vi "gyro -- launch async pll.vi"(8 "pll parameters":T1={"PID parameters"={"I (sec)"=0.004634123928756344, "P (sec)"=0.008980860327047186}, "PID mode"=enum."normal", "lorentzian"={"A (VHz)"=0.0007250653088846297, "f (Hz)"=45017.43809779818, "G (Hz)"=34.46000858512321, "phi(rad)"=-1.525051560312372, "Q"=1306.3675821959234, "Norm  Ampl"=nan, "bg (V)"=7.168586400274938e-06+0.00021232547061132137i, "4corners"={"z (-pi/2)"=-1.288800856206544e-05+0.00019034453621736468i, "z(inf)"=7.168586400274938e-06+0.00021232547061132137i, "z (pi/2)"=-1.4812347993681768e-05+0.00023238206557366173i, "z center"=-1.3850178277873603e-05+0.0002113633008955132i, "z(0)"=-3.486894295602214e-05+0.00021040113117970505i, "radius"=2.1040775631078887e-05}}, "plot hist time (sec)"=1.0, "dt (sec)"=0.001, "visc hist time (sec)"=2.0, "time int ave time (sec)"=0.3, "PLL limits (Hz)"=5000.0, "PLL ON"=FALSE} {"PLL limits (Hz)" format="%#.2f"; "time int ave time (sec)" format="%#_10f"; "visc hist time (sec)" format="%#_10f"; "dt (sec)" format="%#_10f"; "plot hist time (sec)" format="%#_10f"; "lorentzian"."bg (V)" format="%#9_9f"; "lorentzian"."Q" format="%#9_9f"; "lorentzian"."phi(rad)" format="%#9_9f"; "lorentzian"."G (Hz)" format="%#9_9f"; "lorentzian"."f (Hz)" format="%#9_9f"; "PID parameters"."P (sec)" scale=0.01..10.0; "PID parameters"."I (sec)" scale=0.01..10.0}, 10 "talkback event":refnum<user-event>) -> (2 "reference out":refnum<vi>)   [LabVIEW 2018]
uses:
  pll talkback message type.ctl
  pll talkto event type.ctl
  pid -- parameters.ctl
  PID - mode.ctl
  circle corners.ctl
  lorentzian.ctl
  pll parameters.ctl
  pll talkback event.ctl
  pll talkto event.ctl
panel:
  in  "pll talkto event":refnum<vi>
  in  "set step !":dbl(slide)=7372.340425531916 min=0.0 max=16000.0 scale=0.0..16500.0 scale format="%^#6_6g"
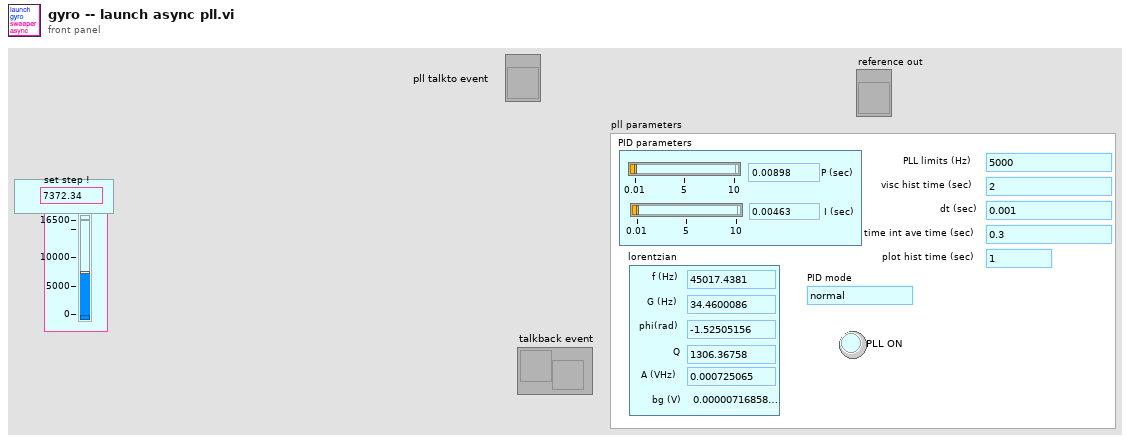
[diagram p1: front panel]
types:
  T1 = typedef "pll parameters.ctl" = cluster{"PID parameters":T2, "PID mode":T3, "lorentzian":T4, "plot hist time (sec)":dbl, "dt (sec)":dbl, "visc hist time (sec)":dbl, "time int ave time (sec)":dbl, "PLL limits (Hz)":dbl, "PLL ON":bool}
  T2 = typedef "pid -- parameters.ctl" = cluster{"I (sec)":dbl, "P (sec)":dbl}
  T3 = typedef "PID - mode.ctl" = enum16{"normal", "heat"}
  T4 = typedef "lorentzian.ctl" = cluster{"A (VHz)":dbl, "f (Hz)":dbl, "G (Hz)":dbl, "phi(rad)":dbl, "Q":dbl, "Norm  Ampl":dbl, "bg (V)":cdb, "4corners":T5}
  T5 = typedef "circle corners.ctl" = cluster{"z (-pi/2)":cdb, "z(inf)":cdb, "z (pi/2)":cdb, "z center":cdb, "z(0)":cdb, "radius":dbl}
  T6 = typedef "pll talkto event type.ctl" = cluster{"message":enum16{"exit", "parameter change", "start", "stop", "reset frequency", "reset lorentzian"}}
  T7 = typedef "pll talkback message type.ctl" = cluster{"message":enum16{"new", ""}}
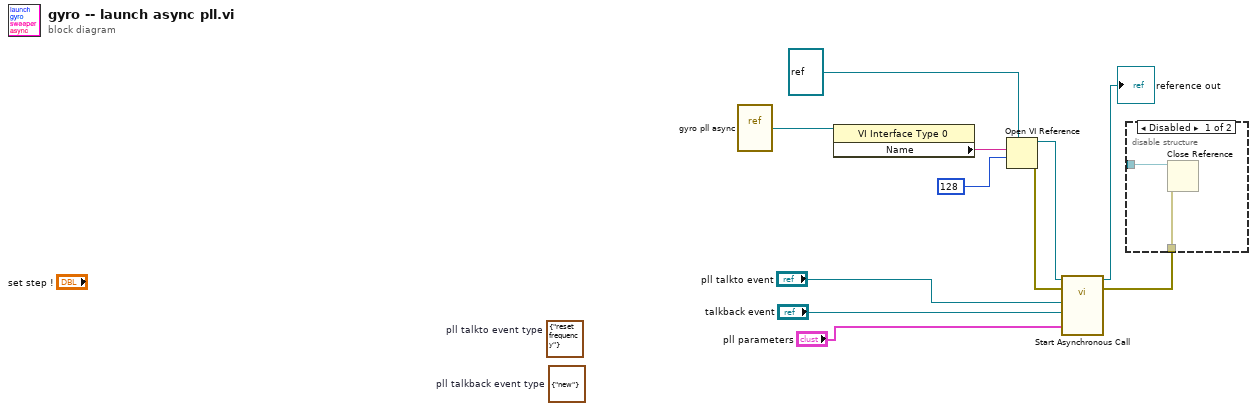
[diagram p0: block diagram]
diagram:
  (unwired) T6 {"message"=enum."reset frequency"}  # pll talkto event type
  (unwired) T7 {"message"=enum."new"}  # pll talkback event type
  n1 = vi-ref "gyro pll async.vi"() -> (w10:refnum<vi>)
  n2 = property class="VI Interface Type 0"(reference=w10) -> ("Name"=w9:string)  [unwired: 1 in, 2 out]
  n3 = Open VI Reference(type specifier VI Refnum (for type only)=refnum<vi> refnum, vi path=w9, options=128) -> (vi reference=w2:refnum<vi>, error out=w7:errorcluster)  [unwired: 3 in]
  n4 = call-by-ref "Start Asynchronous Call"(reference=w2, error in=w7, "pll parameters"="pll parameters", "talkback event"="talkback event", "talkto event"="pll talkto event") -> (reference out=→"reference out":refnum<vi>, error out=w6:errorcluster)  [unwired: 9 in]
  n5 = disable-structure shown="Disabled" {
    disable-tunnel: w6 -> [w13 _]
    disable-tunnel: _ -> [w12 _]
    frame Disabled {
      n6 = Close Reference(reference=w12, error in (no error)=w13) -> ()  [unwired: 1 out]
    }
    frame Enabled {
    }
  }
